vi "arrayToGrayIm.vi"(8 "error in (no error)":errorcluster, 10 "u32 buffer":u32[][](array[numeric]), 11 "Image":T1) -> (0 "error out":errorcluster, 3 "Image Out":T1)   [LabVIEW 2010]
uses:
  <vilib>/vision/Image Controls.llb/IMAQ Image.ctl
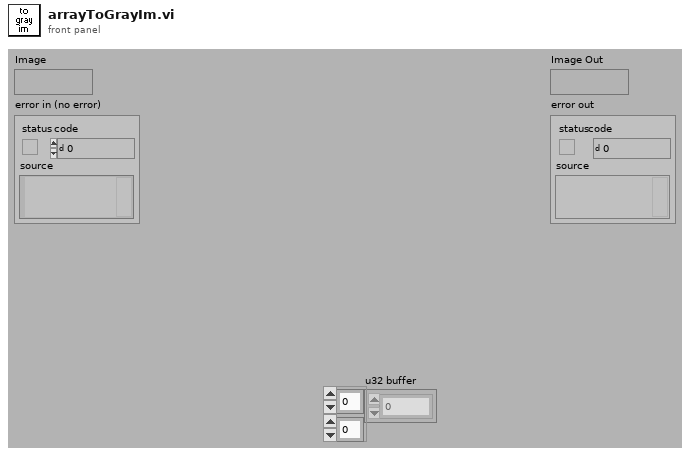
[diagram p1: front panel]
types:
  T1 = typedef "IMAQ Image.ctl" = refnum<image>
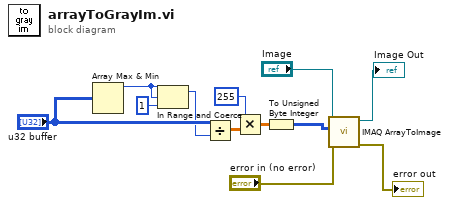
[diagram p0: block diagram]
diagram:
  n1 = Array Max & Min(array="u32 buffer") -> (max value=w1:u32)  [unwired: 3 out]
  n2 = In Range and Coerce(upper limit=w1, x=w1, lower limit=u32 1) -> (coerced(x)=w3:u32)  [unwired: 1 out]
  n3 = Divide(x="u32 buffer", y=w3) -> (x/y=w12:dbl[][])
  n4 = Multiply(x=255, y=w12) -> (x*y=w10:dbl[][])
  n5 = To Unsigned Byte Integer(number=w10) -> (unsigned 8bit integer=w8:u8[][])
  n6 = call "IMAQ ArrayToImage"("error in (no error)"="error in (no error)", "Image Pixels (U8)"=w8, "Image"="Image") -> ("error out"=→"error out":errorcluster, "Image Out"=→"Image Out":T1)  [unwired: 7 in]
